vi "Zaber A move 1 step.vi"(4 "Minimum":dbl, 5 "Maximum":dbl=819200.0, 6 "Direction":enum16{"Forward", "Backward"}(ring), 7 "Device and Axis":string, 8 "error in (no error)":errorcluster, 9 "Current position in":dbl, 10 "Step Size":i32, 11 "VISA Refnum in":refnum<visa-resource-name>) -> (0 "error out":errorcluster, 2 "Position":dbl, 3 "VISA Refnum out":refnum<visa-resource-name>)   [LabVIEW 2013]
uses:
  Drivers and libraries/Zaber A Series/Zaber A Series.lvlib
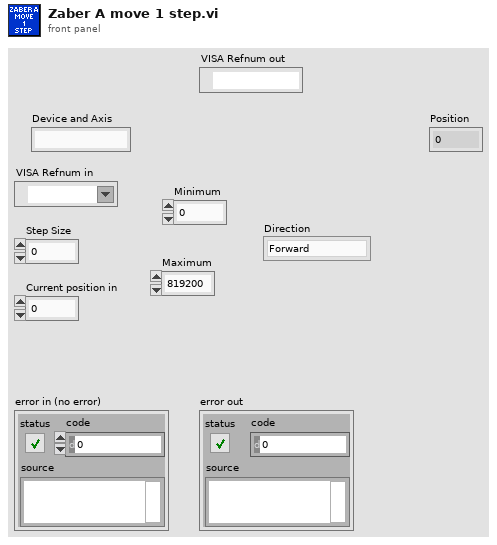
[diagram p1: front panel]
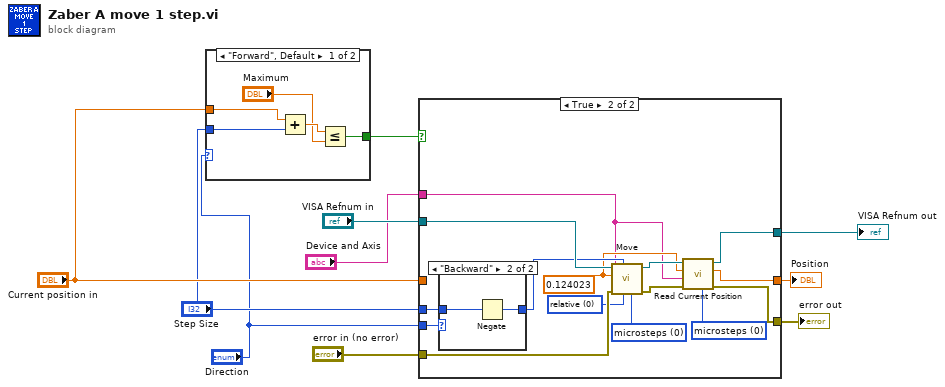
[diagram p0: block diagram]
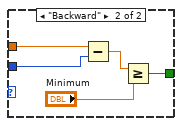
[diagram p2: hidden frame]
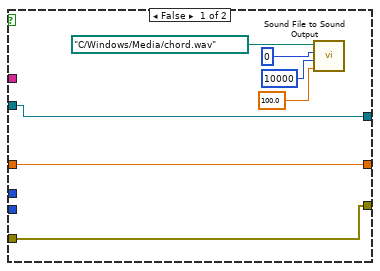
[diagram p3: hidden frame]
diagram:
  n1 = case shown="\"Forward\", Default" "Direction" {
    tunnel: "Current position in" -> [w12 w20]
    tunnel: [w13 w19] -> w9
    tunnel: "Step Size" -> [w14 w17]
    frame "Forward", Default {
      n2 = Add(x=w12, y=w14) -> (x+y=w15:dbl)
      n3 = Less Or Equal?(x=w15, y="Maximum") -> (x <= y?=w13:bool)
    }
    frame "Backward" {
      n4 = Subtract(x=w20, y=w17) -> (x-y=w18:dbl)
      n5 = Greater Or Equal?(x=w18, y="Minimum") -> (x >= y?=w19:bool)
    }
  }
  n6 = case shown="True" w9 {
    tunnel: "Step Size" -> [_ w42]
    tunnel: "VISA Refnum in" -> [w22 w40]
    tunnel: [w27 w30] -> w4
    tunnel: [w22 w29] -> w6
    tunnel: "error in (no error)" -> [w27 w39]
    tunnel: [w21 w28] -> w1
    tunnel: "Current position in" -> [w21 _]
    tunnel: "Direction" -> [_ w41]
    tunnel: "Device and Axis" -> [_ w32]
    frame False {
      n7 = call "Sound File to Sound Output.vi"("Volume"=100.0, "Number of Samples/Iteration"=10000, "Device ID"=u32 0, "File Path"=path "C:/Windows/Media/chord.wav") -> ()
    }
    frame True {
      w31 = u16 0 items=["microsteps", "microns", "millimeters", "inches"] ("Units (0: microsteps)")
      w37 = u16 0 items=["microsteps", "microns", "millimeters", "inches"] ("Units (0: microsteps)")
      w38 = u16 0 items=["relative", "absolute"] ("Movement Type (0: relative)")
      w33 = 0.124023 ("Microstep Size (0)")
      n8 = case shown="\"Backward\"" w41 {
        tunnel: [w43 w45] -> w36
        tunnel: w42 -> [w43 w44]
        frame "Forward", Default {
        }
        frame "Backward" {
          n9 = Negate(x=w44) -> (-x=w45:i32)
        }
      }
      n10 = call "Move.vi"("Units (0: microsteps)"=w37, "Movement Type (0: relative)"=w38, "Move Distance (0)"=w36, "error in (no error)"=w39, "Device and Axis"=w32, "Microstep Size (0)"=w33, "VISA resource name"=w40) -> ("error out"=w34:errorcluster, "VISA resource name out"=w35:refnum<visa-resource-name>)  [unwired: 3 in]
      n11 = call "Read Current Position.vi"("Units (0: microsteps)"=w31, "error in (no error)"=w34, "Device and Axis"=w32, "Microstep Size (0)"=w33, "VISA resource name"=w35) -> ("error out"=w30:errorcluster, "Position"=w28:dbl, "VISA resource name out"=w29:refnum<visa-resource-name>)  [unwired: 4 in]
    }
  }
  "VISA Refnum out" <- w6
  "error out" <- w4
  "Position" <- w1
